vi "_Read.vi"(8 "error in (no error)":errorcluster, 10 "Count":i32, 11 "StringStream in":refnum<class "StringStream.lvclass">) -> (0 "error out":errorcluster, 2 "Data":string, 3 "StringStream out":refnum<class "StringStream.lvclass">)   [LabVIEW 2020, in "Stream.lvlib" / "StringStream.lvclass"]
uses:
  StringStream.lvclass
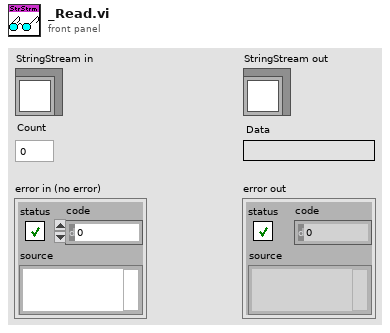
[diagram p1: front panel]
types:
  T1 = typedef "Stream.lvlib/StringStream.lvclass/Ref Data.ctl" = cluster{"Position":i64, "String":string}
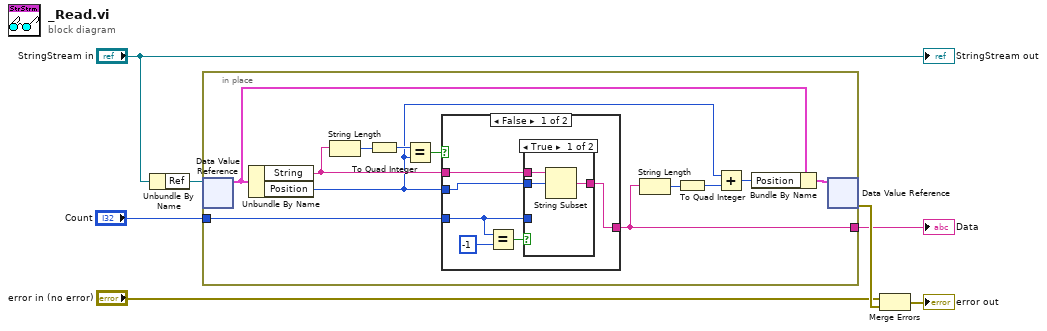
[diagram p0: block diagram]
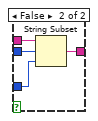
[diagram p2: hidden frame]
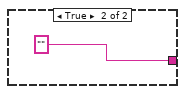
[diagram p3: hidden frame]
diagram:
  n1 = Unbundle By Name("StringStream in") -> ("Ref"=w5:refnum<data-value>)
  n2 = in-place {
    in-place-border: "Count" -> [w16]
    in-place-border: [w14] -> w2
    n3 = in-place-dvr #1(w5) -> (w10:T1)  [unwired: 1 out]
    n4 = Unbundle By Name(w10) -> ("String"=w15:string, "Position"=w12:i64)
    n5 = String Length(string=w15) -> (length=w19:i32)
    n6 = To Quad Integer(1:w19) -> (0:w18:i64)
    n7 = Equal?(x=w18, y=w12) -> (x = y?=w17:bool)
    n8 = case shown="False" w17 {
      tunnel: w16 -> [w21 _]
      tunnel: [w20 ""] -> w14
      tunnel: w15 -> [w25 _]
      tunnel: w12 -> [w24 _]
      frame False {
        n9 = Equal?(x=w21, y=-1) -> (x = y?=w22:bool)
        n10 = case shown="True" w22 {
          tunnel: w25 -> [w28 w32]
          tunnel: w24 -> [w27 w31]
          tunnel: w21 -> [_ w30]
          tunnel: [w26 w29] -> w20
          frame True {
            n11 = String Subset(string=w28, offset (0)=w27) -> (substring=w26:string)  [unwired: 1 in]
          }
          frame False {
            n12 = String Subset(string=w32, offset (0)=w31, length (rest)=w30) -> (substring=w29:string)
          }
        }
      }
      frame True {
      }
    }
    n13 = String Length(string=w14) -> (length=w13:i32)
    n14 = To Quad Integer(1:w13) -> (0:w11:i64)
    n15 = Add(x=w12, y=w11) -> (x+y=w9:i64)
    n16 = Bundle By Name(cluster=w10, "Position"=w9) -> (w8:T1)
    n17 = in-place-dvr #1(w8) -> (w7:errorcluster)  [unwired: 1 out]
  }
  "Data" <- w2
  n18 = Merge Errors("error in (no error)", w7) -> (→"error out":errorcluster)
  "StringStream out" <- "StringStream in"
